vi "Initialize Attributes.vi"(8 "error in (no error)":errorcluster, 10 "Attribute Data":variant, 11 "BNT_DAQmx-MCSV-DOPWM in":refnum<class "BNT_DAQmx-MCSV-DOPWM.lvclass">) -> (0 "error out":errorcluster, 2 "MandatoryParameters":cluster{"Parameter":string, "found?":bool}[](array[cluster]), 3 "BNT_DAQmx-MCSV-DOPWM out":refnum<class "BNT_DAQmx-MCSV-DOPWM.lvclass">)   [LabVIEW 2017, in "BNT_DAQmx.lvlib" / "BNT_DAQmx-MCSV-DOPWM.lvclass"]
doc: "Initialize object attribute.\n\nUnique resources should be allocated elsewhere!"
uses:
  BNT_DAQmx-MCSV-DOPWM.lvclass
  C:/User/Brand/LVP/Acc/VacuumHeating/Packages/CSPP_Core/Actors/CSPP_BaseActor/CSPP_BaseActor.lvclass
  CSPP_Core/Actors/CSPP_BaseActor/CSPP_BaseActor.lvclass/CSPP_BaseActor.ctl
  BNT_DAQmx-MCSV-DOPWM.lvclass/BNT_DAQmx-MCSV-DOPWM.ctl
  BNT_DAQmx-MCSV/BNT_DAQmx-MCSV.lvclass
  CSPP_Core/Classes/CSPP_BaseClasses/Factory/CSPP_Factory.lvclass
  CSPP_Core/Actors/CSPP_BaseActor/CSPP_BaseActor.lvclass
  CSPP_Core/Classes/CSPP_ProcessVariables/CSPP_ProcessVariables.lvlib
  CSPP_Core/Libraries/Utilities/CSPP_Utilities.lvlib
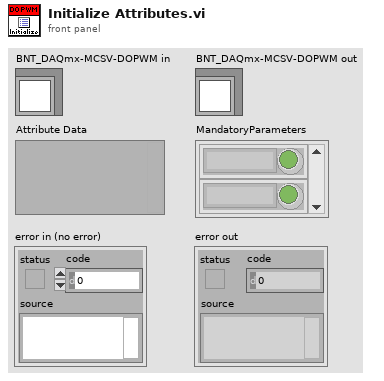
[diagram p1: front panel]
types:
  T1 = cluster{string, "Type Descriptor":string, string}
  T2 = cluster{"initial string":string, "Type Descriptor":string, string}
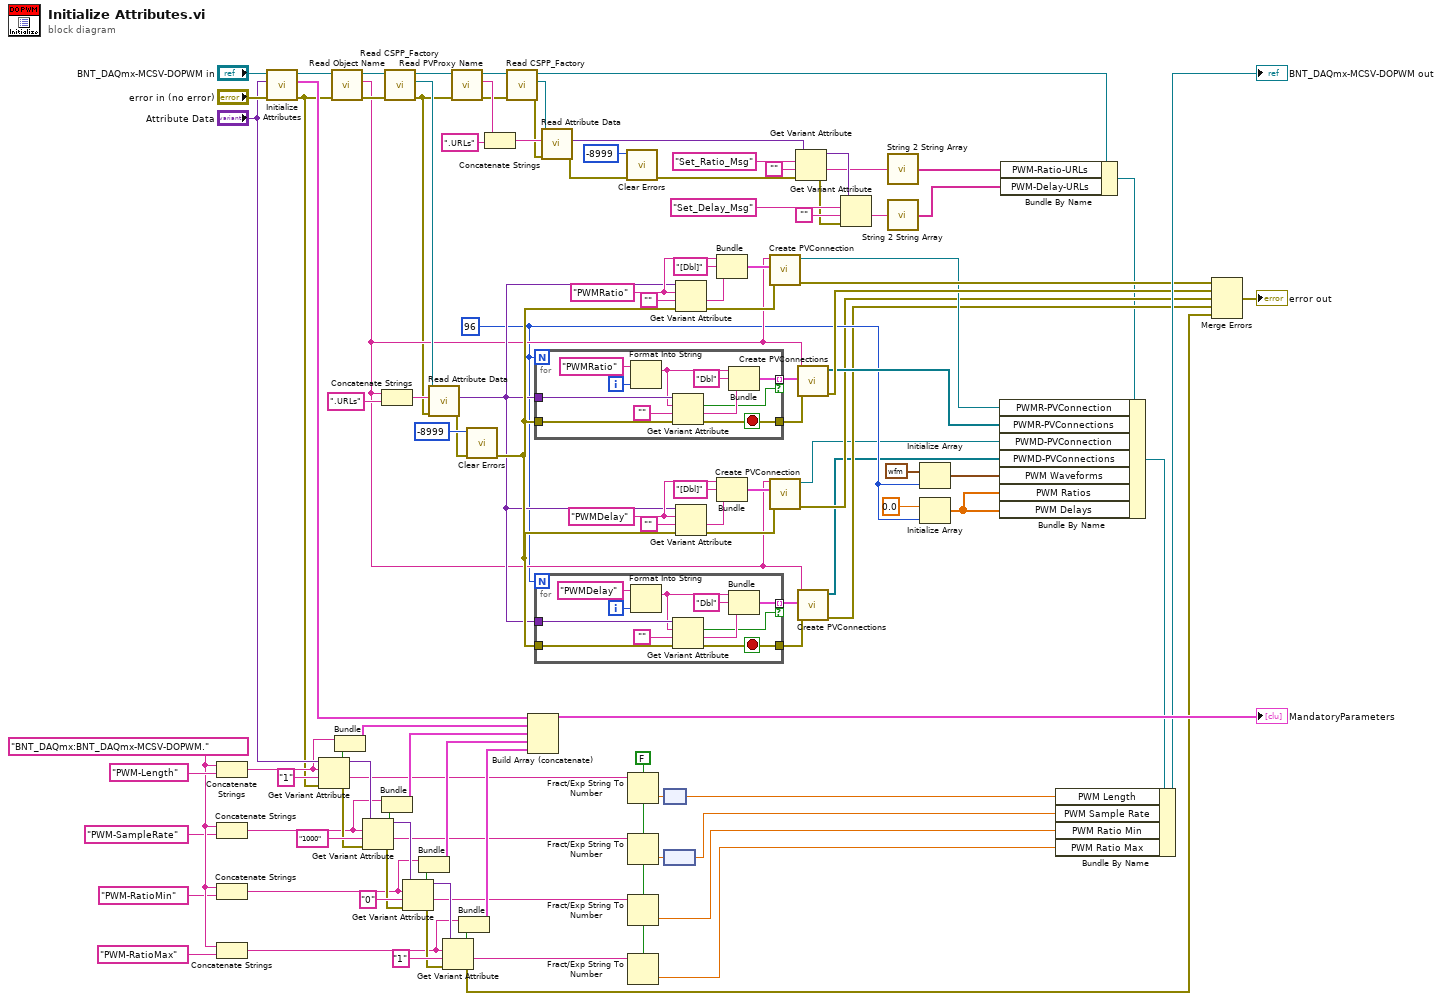
[diagram p0: block diagram]
diagram:
  w39 = "PWMDelay" ("initial string")
  w53 = "PWMRatio" ("initial string")
  w31 = 96
  w57 = FALSE ("use system decimal point (T)")
  w100 = "BNT_DAQmx:BNT_DAQmx-MCSV-DOPWM."
  n1 = Concatenate Strings(w100, "PWM-Length" ("string")) -> (w107:string)
  n2 = Concatenate Strings(w100, "PWM-SampleRate" ("string")) -> (w89:string)
  n3 = Concatenate Strings(w100, "PWM-RatioMin" ("string")) -> (w88:string)
  n4 = Concatenate Strings(w100, "PWM-RatioMax" ("string")) -> (w86:string)
  n5 = call-parent "Initialize Attributes.vi"("error in (no error)"="error in (no error)", "Attribute Data"="Attribute Data", "BNT_DAQmx-MCSV in"="BNT_DAQmx-MCSV-DOPWM in") -> ("error out"=w62:errorcluster, "MandatoryParameters"=w113:cluster{"Parameter":string, "found?":bool}[], "BNT_DAQmx-MCSV out"=w63:refnum<class "BNT_DAQmx-MCSV-DOPWM.lvclass">)  [unwired: 6 in]
  n6 = Get Variant Attribute(Variant="Attribute Data", name=w107, default value (empty Variant)="1" ("string"), error in=w62) -> (duplicate Variant=w96:variant, found=w106:bool, value=w81:string, error out=w95:errorcluster)
  n7 = call "Read Object Name.vi"("error in (no error)"=w62, "CSPP_BaseActor in"=w63) -> ("error out"=w64:errorcluster, "Object Name"=w32:string, "CSPP_BaseActor out"=w70:refnum<class "BNT_DAQmx-MCSV-DOPWM.lvclass">)  [unwired: 7 in]
  n8 = Bundle(w107, w106) -> (w105:cluster{string, bool})  [unwired: 1 in]
  n9 = Get Variant Attribute(Variant=w96, name=w89, default value (empty Variant)="1000" ("string"), error in=w95) -> (duplicate Variant=w94:variant, found=w90:bool, value=w76:string, error out=w93:errorcluster)
  n10 = Concatenate Strings(w32, ".URLs" ("string")) -> (w68:string)
  n11 = Bundle(w89, w90) -> (w84:cluster{string, bool})  [unwired: 1 in]
  n12 = call "Read CSPP_Factory.vi"("error in (no error)"=w64, "CSPP_BaseActor in"=w70) -> ("error out"=w6:errorcluster, "CSPP_Factory"=w65:refnum<class "CSPP_Factory.lvclass">, "CSPP_BaseActor out"=w7:refnum<class "BNT_DAQmx-MCSV-DOPWM.lvclass">)  [unwired: 7 in]
  n13 = Get Variant Attribute(Variant=w94, name=w88, default value (empty Variant)="0" ("string"), error in=w93) -> (duplicate Variant=w92:variant, found=w87:bool, value=w75:string, error out=w91:errorcluster)
  n14 = Bundle(w88, w87) -> (w83:cluster{string, bool})  [unwired: 1 in]
  n15 = call-dynamic "Read Attribute Data.vi"("error in (no error)"=w6, "Object Name"=w68, "CSPP_Factory in"=w65) -> ("error out"=w66:errorcluster, "Attribute Data"=w33:variant)  [unwired: 6 in, 1 out]
  n16 = Get Variant Attribute(Variant=w92, name=w86, default value (empty Variant)="1" ("string"), error in=w91) -> (found=w85:bool, value=w74:string, error out=w58:errorcluster)  [unwired: 1 out]
  n17 = call "Read PVProxy Name.vi"("error in (no error)"=w6, "CSPP_BaseActor in"=w7) -> ("error out"=w8:errorcluster, "PVProxy Name"=w21:string, "CSPP_BaseActor out"=w10:refnum<class "BNT_DAQmx-MCSV-DOPWM.lvclass">)  [unwired: 7 in]
  n18 = Bundle(w86, w85) -> (w82:cluster{string, bool})  [unwired: 1 in]
  n19 = call <vilib>:"Clear Errors.vi"("error in (no error)"=w66, "specific error code to clear (0: all)"=-8999) -> ("error out"=w34:errorcluster)  [unwired: 4 in, 1 out]
  n20 = Concatenate Strings(w21, ".URLs" ("string")) -> (w23:string)
  n21 = call "Read CSPP_Factory.vi"("error in (no error)"=w8, "CSPP_BaseActor in"=w10) -> ("error out"=w5:errorcluster, "CSPP_Factory"=w9:refnum<class "CSPP_Factory.lvclass">, "CSPP_BaseActor out"=w4:refnum<class "BNT_DAQmx-MCSV-DOPWM.lvclass">)  [unwired: 7 in]
  n22 = Build Array (concatenate)(w113, w105, w84, w83, w82) -> (→"MandatoryParameters":cluster{"Parameter":string, "found?":bool}[])
  n23 = for {
    N: w31 -> [_]
    tunnel: w33 -> [w123]
    tunnel: w34 -> [w122]
    tunnel: [w118] -> w61 mode=indexing if=w115
    tunnel: [w114] -> w60
    i -> [w121]
    stop <- w114 stop-if-true
    n24 = Format Into String(initial string="PWMRatio", w121) -> (resulting string=w119:string)  [unwired: 2 in, 1 out]
    n25 = Get Variant Attribute(Variant=w123, name=w119, default value (empty Variant)="", error in=w122) -> (found=w115:bool, value=w116:string, error out=w114:errorcluster)  [unwired: 1 out]
    n26 = Bundle(w119, "Type Descriptor"="Dbl", w116) -> (w118:T1)  [unwired: 1 in]
  }
  n27 = for {
    N: w31 -> [_]
    tunnel: w33 -> [w134]
    tunnel: w34 -> [w133]
    tunnel: [w129] -> w35 mode=indexing if=w126
    tunnel: [w125] -> w36
    i -> [w132]
    stop <- w125 stop-if-true
    n28 = Format Into String(initial string="PWMDelay", w132) -> (resulting string=w130:string)  [unwired: 2 in, 1 out]
    n29 = Get Variant Attribute(Variant=w134, name=w130, default value (empty Variant)="", error in=w133) -> (found=w126:bool, value=w127:string, error out=w125:errorcluster)  [unwired: 1 out]
    n30 = Bundle(w130, "Type Descriptor"="Dbl", w127) -> (w129:T1)  [unwired: 1 in]
  }
  n31 = call-dynamic "Read Attribute Data.vi"("error in (no error)"=w5, "Object Name"=w23, "CSPP_Factory in"=w9) -> ("error out"=w25:errorcluster, "Attribute Data"=w19:variant)  [unwired: 6 in, 1 out]
  n32 = call <vilib>:"Clear Errors.vi"("error in (no error)"=w25, "specific error code to clear (0: all)"=-8999) -> ("error out"=w18:errorcluster)  [unwired: 4 in, 1 out]
  n33 = Fract/Exp String To Number(use system decimal point (T)=w57, string=w81) -> (number=w79:dbl)  [unwired: 2 in, 1 out]
  n34 = Fract/Exp String To Number(use system decimal point (T)=w57, string=w76) -> (number=w77:dbl)  [unwired: 2 in, 1 out]
  n35 = Fract/Exp String To Number(use system decimal point (T)=w57, string=w75) -> (number=w72:dbl)  [unwired: 2 in, 1 out]
  n36 = Fract/Exp String To Number(use system decimal point (T)=w57, string=w74) -> (number=w71:dbl)  [unwired: 2 in, 1 out]
  n37 = node(w79) -> (w78:dbl[unit])
  n38 = node(w77) -> (w73:dbl[unit])
  n39 = Get Variant Attribute(Variant=w33, name=w53, default value (empty Variant)="", error in=w34) -> (value=w52:string, error out=w50:errorcluster)  [unwired: 2 out]
  n40 = Get Variant Attribute(Variant=w33, name=w39, default value (empty Variant)="", error in=w34) -> (value=w40:string, error out=w42:errorcluster)  [unwired: 2 out]
  n41 = Bundle("initial string"=w53, "Type Descriptor"="[Dbl]", w52) -> (w51:T2)  [unwired: 1 in]
  n42 = Bundle("initial string"=w39, "Type Descriptor"="[Dbl]", w40) -> (w41:T2)  [unwired: 1 in]
  n43 = call "Create PVConnection.vi"("Error In"=w50, "PV-Info"=w51, "Object Name"=w32) -> ("error out"=w49:errorcluster, "PVConnection"=w45:refnum<class "PVConnection.lvclass">)  [unwired: 7 in]
  n44 = call "Create PVConnection.vi"("Error In"=w42, "PV-Info"=w41, "Object Name"=w32) -> ("error out"=w30:errorcluster, "PVConnection"=w28:refnum<class "PVConnection.lvclass">)  [unwired: 7 in]
  n45 = Get Variant Attribute(Variant=w19, name="Set_Ratio_Msg", default value (empty Variant)="", error in=w18) -> (duplicate Variant=w14:variant, value=w12:string, error out=w13:errorcluster)  [unwired: 1 out]
  n46 = call "Create PVConnections.vi"("Error In"=w60, "PV-Infos"=w61, "Object Name"=w32) -> ("error out"=w59:errorcluster, "PVConnections"=w44:refnum<class "PVConnection.lvclass">[])  [unwired: 7 in]
  n47 = call "Create PVConnections.vi"("Error In"=w36, "PV-Infos"=w35, "Object Name"=w32) -> ("error out"=w29:errorcluster, "PVConnections"=w27:refnum<class "PVConnection.lvclass">[])  [unwired: 7 in]
  n48 = Get Variant Attribute(Variant=w14, name="Set_Delay_Msg", default value (empty Variant)="", error in=w13) -> (value=w11:string)  [unwired: 3 out]
  n49 = call "String 2 String Array.vi"("String"=w12) -> ("Substrings"=w2:string[])  [unwired: 1 in]
  n50 = call "String 2 String Array.vi"("String"=w11) -> ("Substrings"=w1:string[])  [unwired: 1 in]
  n51 = Initialize Array(waveform(dbl) {"t0"=timestamp(-9593251200 s since 1904-01-01), "dt"=0.001, "Y"=[]} ("PWM Waveform"), w31) -> (w43:waveform(dbl)[])
  n52 = Initialize Array(0.0 ("PWM Ratio"), w31) -> (w26:dbl[])
  n53 = Bundle By Name(cluster=w4, "PWM-Ratio-URLs"=w2, "PWM-Delay-URLs"=w1) -> (w3:refnum<class "BNT_DAQmx-MCSV-DOPWM.lvclass">)
  n54 = Bundle By Name(cluster=w3, "PWMR-PVConnection"=w45, "PWMR-PVConnections"=w44, "PWMD-PVConnection"=w28, "PWMD-PVConnections"=w27, "PWM Waveforms"=w43, "PWM Ratios"=w26, "PWM Delays"=w26) -> (w46:refnum<class "BNT_DAQmx-MCSV-DOPWM.lvclass">)
  n55 = Bundle By Name(cluster=w46, "PWM Length"=w78, "PWM Sample Rate"=w73, "PWM Ratio Min"=w72, "PWM Ratio Max"=w71) -> (→"BNT_DAQmx-MCSV-DOPWM out":refnum<class "BNT_DAQmx-MCSV-DOPWM.lvclass">)
  n56 = Merge Errors(w49, w59, w30, w29, w58) -> (→"error out":errorcluster)
